vi "K-2100 read resistance.vi"() -> ()   [LabVIEW 2014]
uses:
  Environmental Chamber LabVIEW and Instruments/Drivers and Software/Keithley 2100 Series/Public/Configure/Configure 2 Wire Resistance.vi
  Environmental Chamber LabVIEW and Instruments/Drivers and Software/Keithley 2100 Series/Keithley 2100 Series.lvlib
panel:
  out "error out":errorcluster
  out "K-2100 Ohms":dbl
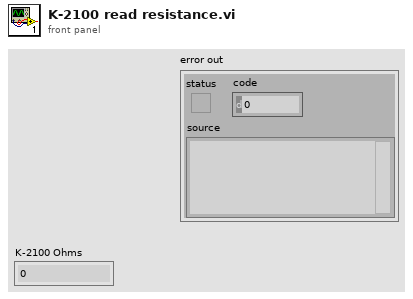
[diagram p1: front panel]
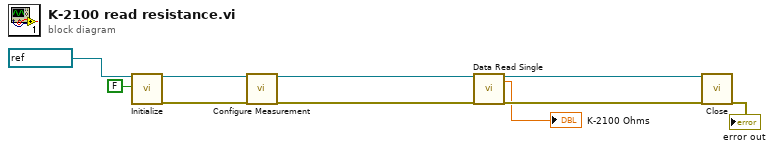
[diagram p0: block diagram]
diagram:
  n1 = call "Initialize.vi"("VISA resource name"=refnum<visa-resource-name> "K-2100", "Reset? (T: Reset)"=FALSE) -> ("VISA resource name out"=w7:refnum<visa-resource-name>, "error out"=w10:errorcluster)  [unwired: 16 in]
  n2 = call-poly "Configure Measurement.vi"("VISA resource name"=w7, "error in (no error)"=w10) -> ("VISA resource name out"=w3:refnum<visa-resource-name>, "error out"=w2:errorcluster)  [unwired: 16 in]
  n3 = call "Data Read Single.vi"("VISA resource name"=w3, "error in (no error)"=w2) -> ("VISA resource name out"=w8:refnum<visa-resource-name>, "Measurement"=→"K-2100 Ohms":dbl, "error out"=w9:errorcluster)  [unwired: 15 in]
  n4 = call "Close.vi"("VISA resource name"=w8, "error in (no error)"=w9) -> ("error out"=→"error out":errorcluster)  [unwired: 17 in]
